vi "SendFileCommand.vi"(8 "error in (no error)":errorcluster, 10 "file data":T1, 11 "Queue in":refnum<queue>) -> (0 "error out":errorcluster, 3 "Queue out":refnum<queue>)   [LabVIEW 2016]
doc: "sends the file data to the data analyzer loop"
uses:
  DataType.ctl
  data_command_enum.ctl
  FileData.ctl
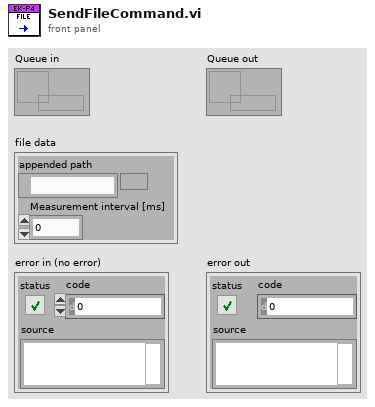
[diagram p1: front panel]
types:
  T1 = typedef "FileData.ctl" = cluster{"appended path":path, "Measurement interval [ms]":u16}
  T2 = typedef "data_command_enum.ctl" = enum16{"data", "display", "quit", "save", "filepath", "weak left", "state", "weak right", "strong left", "strong right", "stopRecording", "close", "sid"}
  T3 = typedef "DataType.ctl" = cluster{"command":T2, "data":variant}
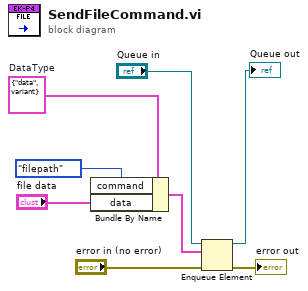
[diagram p0: block diagram]
diagram:
  w5 = T3 {"command"=enum."data", "data"=variant(dbl[] [])}  # DataType
  n1 = Bundle By Name(cluster=w5, "command"=data_command_enum."filepath", "data"="file data") -> (w4:T3)
  n2 = Enqueue Element(queue="Queue in", element=w4, error in (no error)="error in (no error)") -> (queue out=→"Queue out":refnum<queue>, error out=→"error out":errorcluster)  [unwired: 1 in, 1 out]
